vi "Control.vi"(1 "uc IN":T1, 2 "Wire in":T2, 8 "dc IN":T1) -> (4 "uc OUT":T1, 5 "dc OUT":T1, 7 "Wire out":T2)   [LabVIEW 2016]
uses:
  TypeDefs/Circuit Cluster.ctl
  Classes/GateAbst/GateAbst.lvclass
  TypeDefs/Controls.ctl
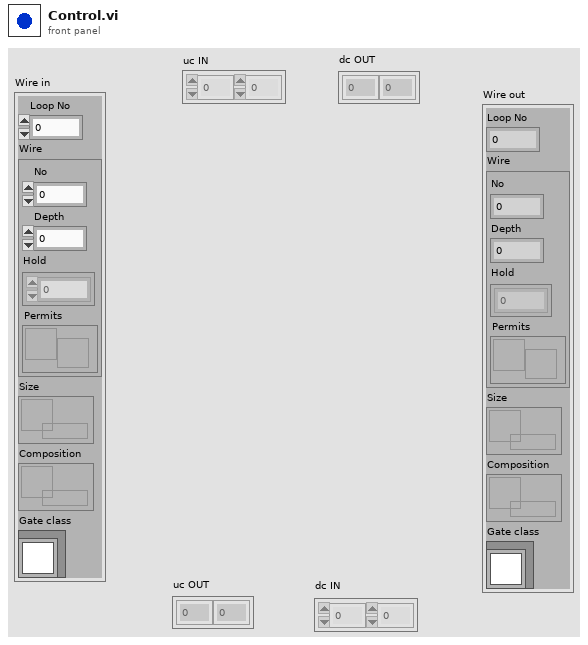
[diagram p1: front panel]
types:
  T1 = typedef "Controls.ctl" = i32[][]
  T2 = typedef "Circuit Cluster.ctl" = cluster{"Loop No":i32, "Wire":cluster{"No":i32, "Depth":i32, "Hold":i32[][], "Permits":refnum<notifier>}, "Size":refnum<queue>, "Composition":refnum<queue>, "Gate class":refnum<class "GateAbst.lvclass">}
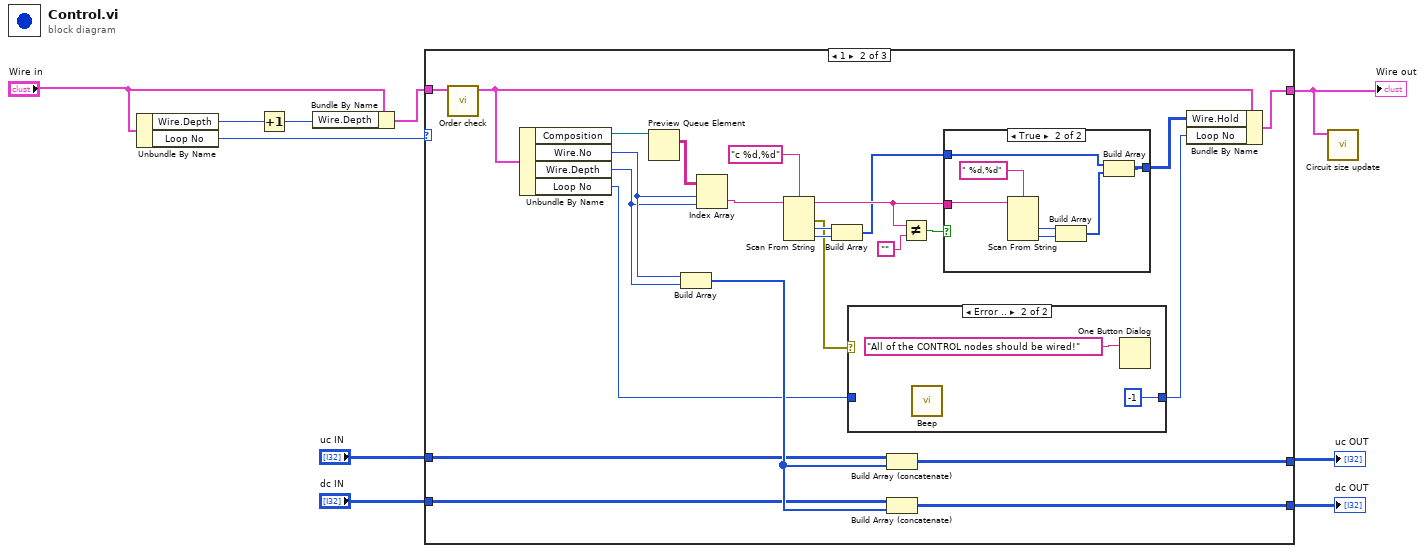
[diagram p0: block diagram]
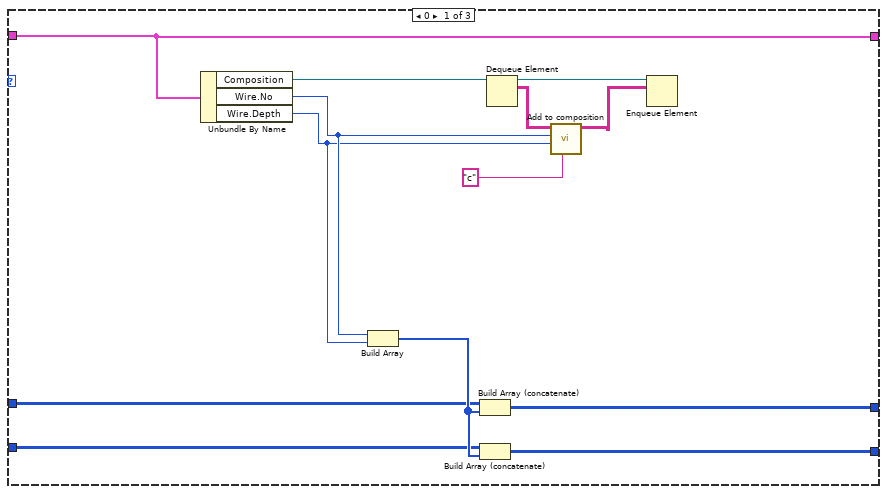
[diagram p2: hidden frame]
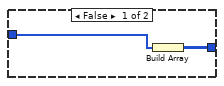
[diagram p4: hidden frame]
diagram:
  n1 = Unbundle By Name("Wire in") -> ("Wire.Depth"=w10:i32, "Loop No"=w1:i32)
  n2 = Increment(x=w10) -> (x+1=w8:i32)
  n3 = Bundle By Name(cluster="Wire in", "Wire.Depth"=w8) -> (w9:T2)
  n4 = case shown="1" w1 {
    tunnel: w9 -> [w11 w26 w62]
    tunnel: [w11 w38 w62] -> w2
    tunnel: "uc IN" -> [w17 w32 w61]
    tunnel: [w16 w31 w61] -> w6
    tunnel: "dc IN" -> [w15 w30 w60]
    tunnel: [w14 w29 w60] -> w4
    frame 0 {
      n5 = Unbundle By Name(w11) -> ("Composition"=w22:refnum<queue>, "Wire.No"=w20:i32, "Wire.Depth"=w19:i32)
      n6 = Build Array(w20, w19) -> (w18:i32[])
      n7 = Build Array (concatenate)(w17, w18) -> (w16:T1)
      n8 = Build Array (concatenate)(w15, w18) -> (w14:T1)
      n9 = Dequeue Element(queue=w22) -> (queue out=w21:refnum<queue>, element=w23:string[][])  [unwired: 2 in, 2 out]
      n10 = call "Add to composition.vi"("Gate name"="c", "Wire depth"=w19, "Wire No"=w20, "Composition in"=w23) -> ("Composition out"=w13:string[][])  [unwired: 7 in]
      n11 = Enqueue Element(queue=w21, element=w13) -> ()  [unwired: 2 in, 3 out]
    }
    frame 1 {
      n12 = call "Order check.vi"("Wire in in"=w26) -> ("Wire out"=w27:T2)  [unwired: 10 in]
      n13 = Unbundle By Name(w27) -> ("Composition"=w43:refnum<queue>, "Wire.No"=w37:i32, "Wire.Depth"=w36:i32, "Loop No"=w25:i32)
      n14 = Preview Queue Element(queue=w43) -> (element=w42:string[][])  [unwired: 2 in, 3 out]
      n15 = Build Array(w37, w36) -> (w35:i32[])
      n16 = Index Array(array=w42, index (row)=w37, index (col)=w36) -> (element=w41:string)
      n17 = Scan From String(format string="c %d,%d", input string=w41) -> (remaining string=w47:string, error out=w28:errorcluster, output 1=w40:i32, output 2=w39:i32)  [unwired: 4 in, 1 out]
      n18 = Build Array(w40, w39) -> (w34:i32[])
      n19 = case shown="Error .." w28 {
        tunnel: w25 -> [w48 _]
        tunnel: [w48 -1 ("Loop No")] -> w24
        frame No Error {
        }
        frame Error {
          n20 = call <vilib>:"Beep.vi"() -> ()  [unwired: 12 in]
          n21 = One Button Dialog(message="All of the CONTROL nodes should be wired!") -> ()  [unwired: 1 in, 1 out]
        }
      }
      n22 = Build Array (concatenate)(w32, w35) -> (w31:T1)
      n23 = Build Array (concatenate)(w30, w35) -> (w29:T1)
      n24 = Not Equal?(x=w47, y="") -> (x != y?=w46:bool)
      n25 = case shown="True" w46 {
        tunnel: w47 -> [_ w58]
        tunnel: w34 -> [w51 w54]
        tunnel: [w52 w53] -> w33
        frame False {
          n26 = Build Array(w51) -> (w52:i32[][])
        }
        frame True {
          n27 = Scan From String(format string=" %d,%d", input string=w58) -> (output 1=w57:i32, output 2=w56:i32)  [unwired: 4 in, 3 out]
          n28 = Build Array(w57, w56) -> (w55:i32[])
          n29 = Build Array(w54, w55) -> (w53:i32[][])
        }
      }
      n30 = Bundle By Name(cluster=w27, "Wire.Hold"=w33, "Loop No"=w24) -> (w38:T2)
    }
    frame Default {
    }
  }
  "Wire out" <- w2
  "uc OUT" <- w6
  "dc OUT" <- w4
  n31 = call "Circuit size update.vi"("Wire in"=w2) -> ()  [unwired: 11 in]
